vi "Send Logging Command.vi"(6 "overwrite on timeout (T)":bool, 8 "error in (no error)":errorcluster, 9 "timeout in ms (0)":i32 format="%d ms", 10 "command":T1={"Command"=enum."Log Framework State", "Parameters"={"arg1"=0, "arg2"=0}}, 11 "Logging Interface in":refnum<class "Logging Interface.lvclass">) -> (0 "error out":errorcluster, 3 "Logging Interface out":refnum<class "Logging Interface.lvclass">)   [LabVIEW 2020, in "DSF Core.lvlib" / "Logging Interface.lvclass"]
uses:
  Logging Interface.lvclass
  Interface.lvclass
  DSF Core.lvlib
  C:/Users/nitest/Desktop/Git/niveristand-data-sharing-framework-custom-device/Source/Core/Classes/Interface/Interface.lvclass
  C:/Users/nitest/Desktop/Git/niveristand-data-sharing-framework-custom-device/Source/Core/Classes/Interface/Logging/Logging Interface.lvclass
  Dispatcher/Command Timeout.vi
  Command.ctl
  Parameters.ctl
  Command Data.ctl
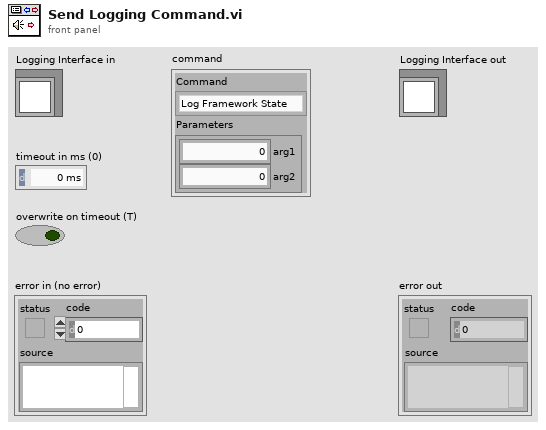
[diagram p1: front panel]
types:
  T1 = typedef "DSF Core.lvlib/Logging Interface.lvclass/Command Data.ctl" = cluster{"Command":T2, "Parameters":T3}
  T2 = typedef "DSF Core.lvlib/Logging Interface.lvclass/Command.ctl" = enum8{"Idle", "Start", "Log Framework State", "Log Plugin State", "Log Dispatcher State", "Shutdown"}
  T3 = typedef "DSF Core.lvlib/Logging Interface.lvclass/Parameters.ctl" = cluster{"arg1":u64, "arg2":u64}
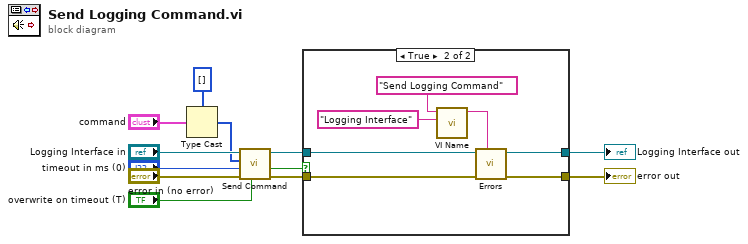
[diagram p0: block diagram]
diagram:
  n1 = Type Cast(type=u8[] [] ("element"), x="command") -> (*(type *) &x=w10:u8[])
  n2 = call "Send Command.vi"("overwrite on timeout (T)"="overwrite on timeout (T)", "error in (no error)"="error in (no error)", "timeout in ms (0)"="timeout in ms (0)", "command data"=w10, "Interface in"="Logging Interface in") -> ("error out"=w6:errorcluster, "timed out?"=w5:bool, "Interface out"=w7:refnum<class "Logging Interface.lvclass">)  [unwired: 3 in, 1 out]
  n3 = case shown="True" w5 {
    tunnel: w6 -> [w13 w20]
    tunnel: w7 -> [w14 w21]
    tunnel: [w14 w19] -> w4
    tunnel: [w13 w18] -> w3
    frame False {
    }
    frame True {
      n4 = call "VI Name.vi"("class name (\"\")"="Logging Interface" ("class name (\"\")"), "vi name"="Send Logging Command" ("error source vi name")) -> ("full VI name"=w16:string)  [unwired: 9 in]
      n5 = call-poly "Errors.vi"("error source vi name"=w16, "error in (no error)"=w20, "Interface in"=w21) -> ("error out"=w18:errorcluster, "Interface out"=w19:refnum<class "Logging Interface.lvclass">)  [unwired: 7 in]
    }
  }
  "error out" <- w3
  "Logging Interface out" <- w4
